vi "Axis Settings.vi"(8 "Updates Per Point":u32, 9 "Ramp":i32, 10 "Offset":i32, 11 "Center Frequency":u32) -> (0 "Falling Rate":u32, 1 "Rising Rate":u32, 2 "Low":u32, 3 "High":u32)   [LabVIEW 2014]
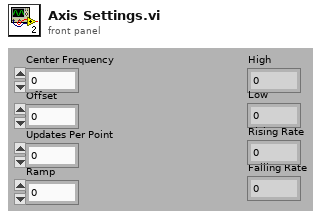
[diagram p1: front panel]
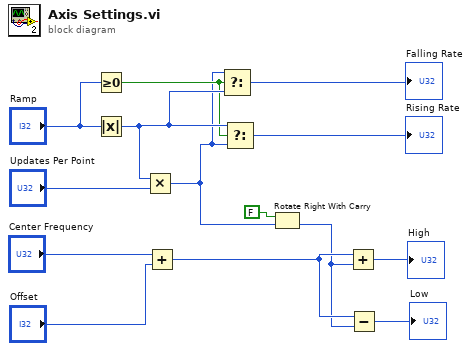
[diagram p0: block diagram]
diagram:
  n1 = Greater Or Equal To 0?(x="Ramp") -> (x >= 0?=w4:bool)
  n2 = Absolute Value(x="Ramp") -> (abs(x)=w5:i32)
  n3 = Multiply(x=w5, y="Updates Per Point") -> (x*y=w1:u32)
  n4 = Add(x="Center Frequency", y="Offset") -> (x+y=w10:u32)
  n5 = Select(t=w1, s=w4, f=w5) -> (s? t:f=→"Falling Rate":u32)
  n6 = Select(t=w5, s=w4, f=w1) -> (s? t:f=→"Rising Rate":u32)
  n7 = Rotate Right With Carry(2:w1, 3:FALSE ("carry")) -> (0:w9:u32)  [unwired: 1 out]
  n8 = Add(x=w10, y=w9) -> (x+y=→"High":u32)
  n9 = Subtract(x=w10, y=w9) -> (x-y=→"Low":u32)
